vi "test_vlp16.vi"() -> ()   [LabVIEW 2019]
uses:
  <vilib>/Utility/miscctls.llb/LV3DPointTypeDef.ctl
  <vilib>/picture/3D Picture Control/Object/Create Object (drawable).vi
  <vilib>/picture/3D Picture Control/Object/Add Object (no reference).vi
  <vilib>/picture/3D Picture Control/Helpers/Set Light (no reference).vi
  <vilib>/picture/3D Picture Control/NI_3D Picture Control.lvlib
panel:
  in  "VLP16 cfg":T1={"h range"={82, -88}, "v range"={7, -9}} {"v range" scale=-15.0..15.0; "h range" scale=-180.0..180.0}
  in  "탭 컨트롤":enum32{"xy graph", "Data"}(tab)
  out "size_vlp-array":i32=12936
  out "3D Picture":refnum<vi>(3d-picture)
  in  "Draw Mode":T2(ring)
  in  "Size":dbl(slide)=1.3265306122448979 scale=0.0..10.0
  out "frame per s":dbl=9.75287984411405 format="%#_2g"
  out "For loop":i32=76
  in  "N of slice":u32=2048
  in  "dt":u32=10
  in  "Enable 3D":bool
  out "XY data":cluster{"x":dbl, "y":dbl}[](graph)
  in  "limit":dbl(slide) scale=0.0..10.0
  out "all_data":T3(array[cluster])
  out "xyz data":cluster{"x":dbl, "y":dbl, "z":dbl}[](array[cluster])
  in  "sel arrary":dbl[](array[numeric])=[-15.0, 1.0, -13.0, 3.0, -11.0, 5.0, -9.0, 7.0, -7.0, 9.0, -5.0, 11.0, -3.0, 13.0, -1.0, 15.0]
  in  "Enable deg":bool[](array[boolean])=[FALSE, TRUE, FALSE, TRUE, FALSE, TRUE, FALSE, FALSE, TRUE, FALSE, TRUE, FALSE, TRUE, FALSE, TRUE, FALSE]
  out "XY Graph":T4(graph)
  out "dt":u32=60
  out "Slide":i16(slide) scale=0.0..1000.0
  in  "stop":bool=TRUE
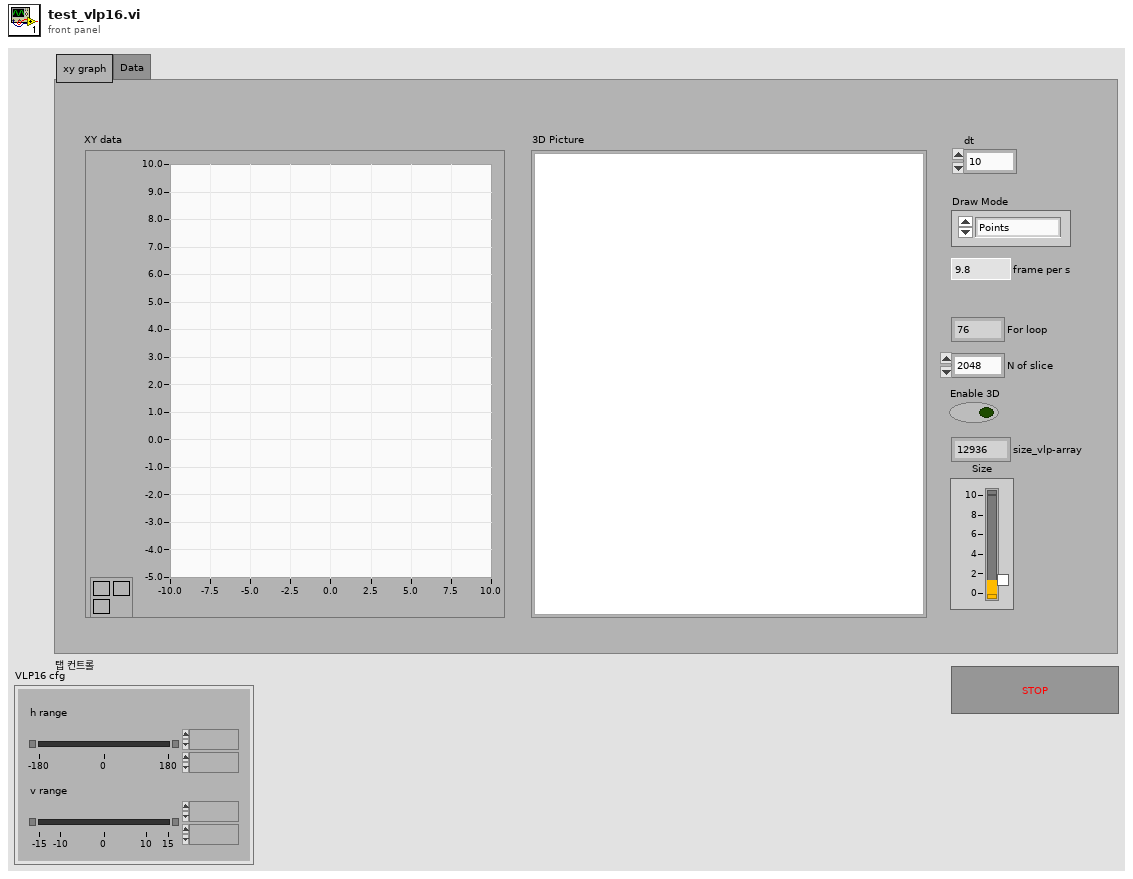
[diagram p1: front panel]
types:
  T1 = cluster{"h range":cluster{i16, i16}, "v range":cluster{i8, i8}}
  T2 = enum16{"Points", "Lines", "Line Strip", "Line Loop", "Triangles", "Triangle Strip", "Triangle Fan", "Quads", "Quad Strip", "Polygon"}
  T3 = cluster{"id":i32, "arimuth(degree)":dbl, "vertical(degree)":dbl, "distance(meter)":dbl, "reflectivity":u8, "times(s)":ext, "x":dbl, "y":dbl, "z":dbl}[]
  T4 = cluster{"Array out":cluster{"x":dbl, "y":dbl}[]}[]
  T5 = enum16{"Inherit Value", "Points", "Wireframe", "Polygons"}
  T6 = typedef "LV3DPointTypeDef.ctl" = cluster{"X":sgl, "Y":sgl, "Z":sgl}
  T7 = cluster{"id":i32, "azimuth(degree)":dbl, "vertical(degree)":dbl, "distance(meter)":dbl, "reflectivity":u8, "time(s)":ext, "x":dbl, "y":dbl, "z":dbl}
  T8 = cluster{"id":i32, "azimuth(degree)":dbl, "vertical(degree)":dbl, "distance(meter)":dbl, "reflectivity":u8, "time(s)":ext, "x":dbl, "y":dbl, "z":dbl}[]
  T9 = cluster{"limit inrange xydata":cluster{"x":dbl, "y":dbl}[]}
  T10 = cluster{"limit inrange xydata":cluster{"x":dbl, "y":dbl}[]}[]
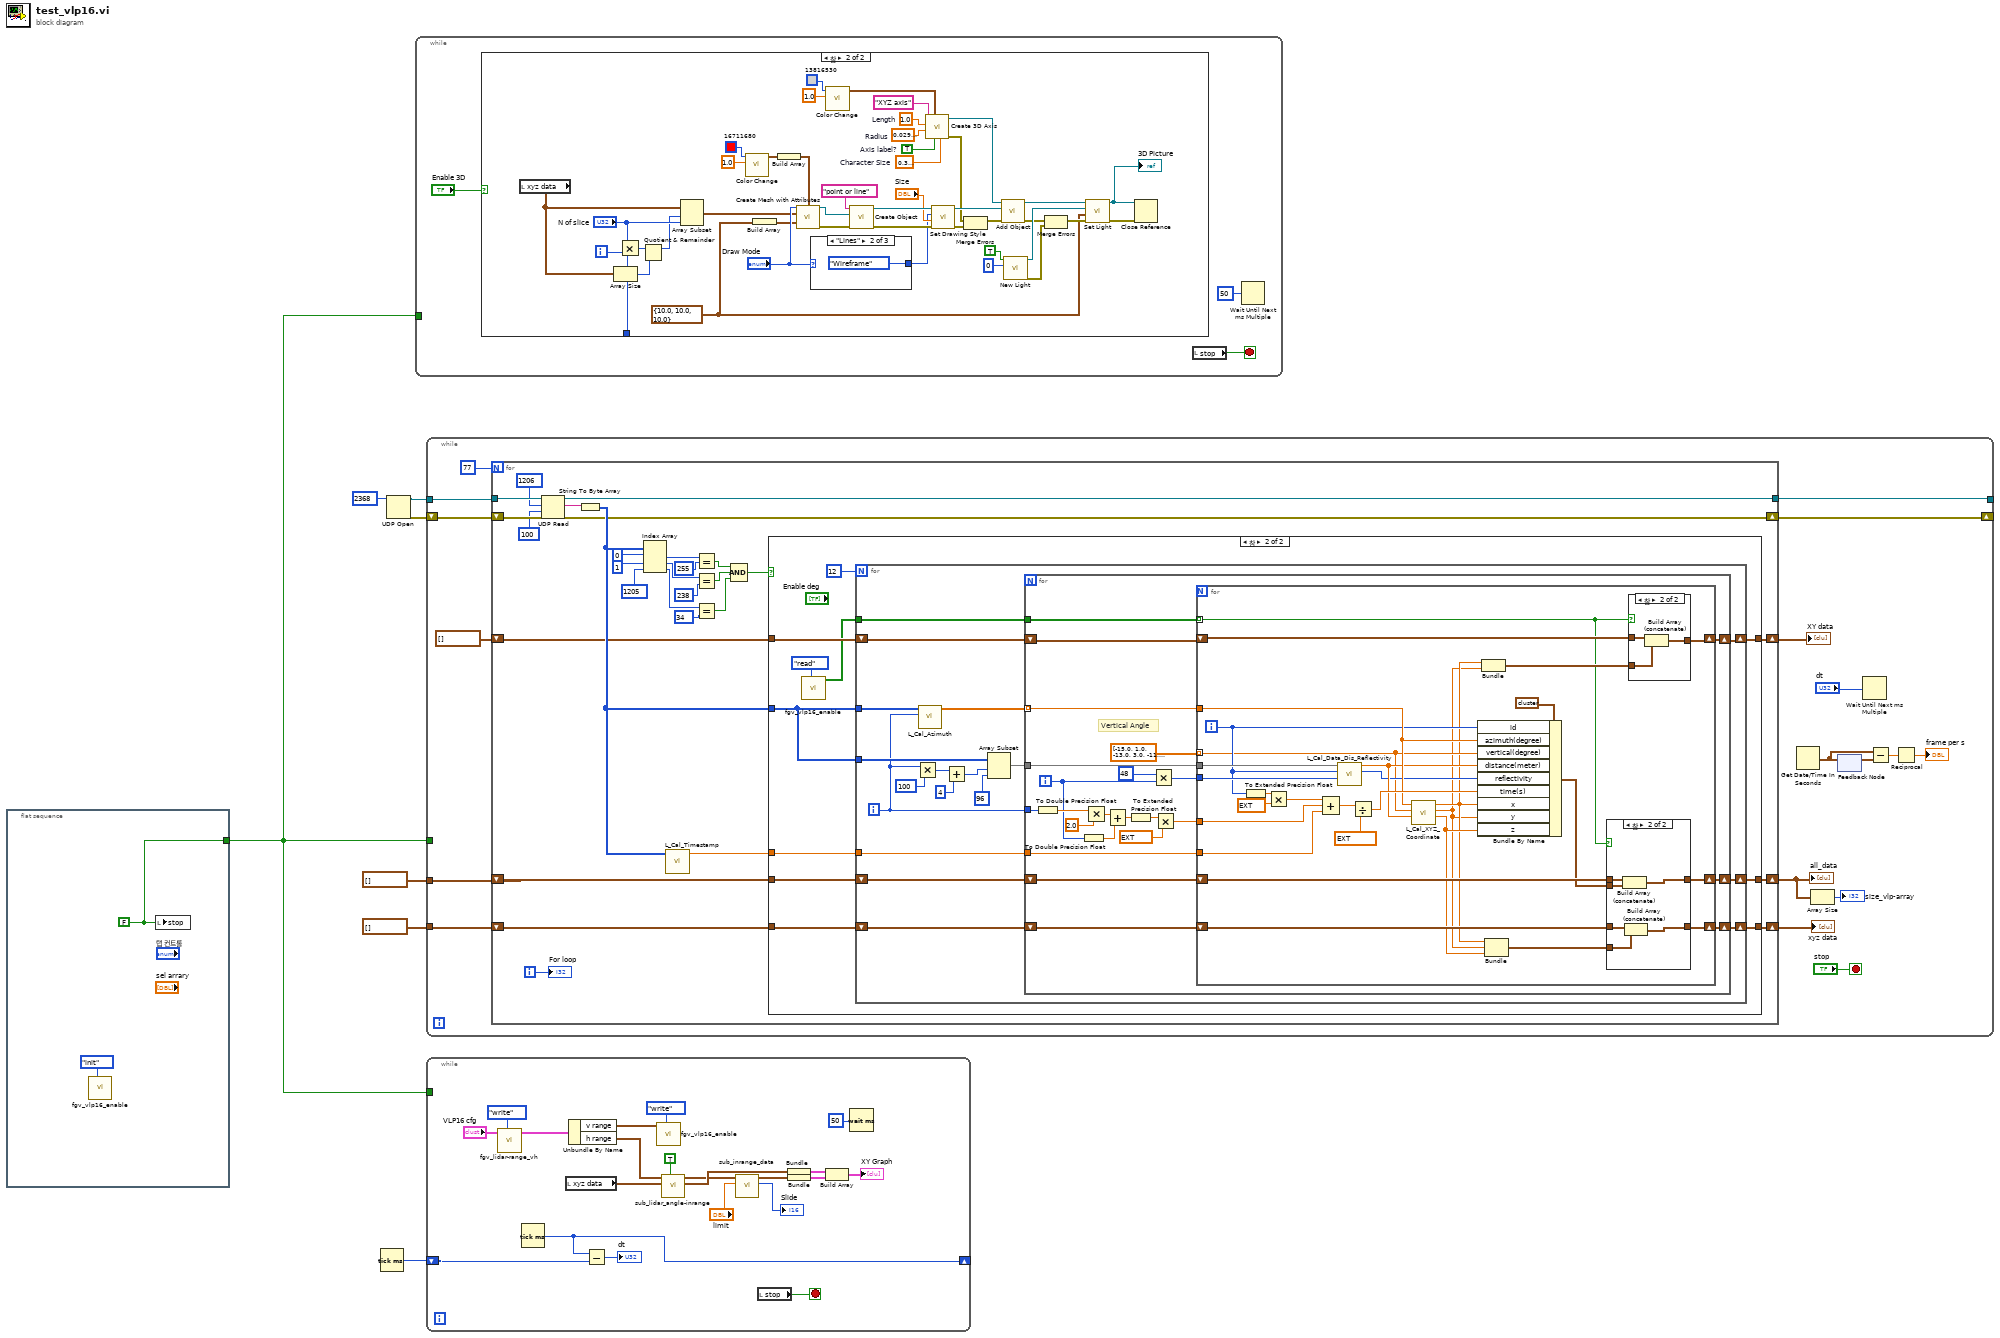
[diagram p0: block diagram]
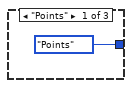
[diagram p3: hidden frame]
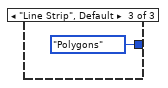
[diagram p4: hidden frame]
diagram:
  n1 = flat-sequence {
    tunnel: [w9] -> w1
    frame #0 {
      w9 = FALSE ("stop")
      n2 = call "fgv_vlp16_enable.vi"("cmd"=enum16{"init", "read", "write"}."init") -> ()  [unwired: 10 in, 1 out]
      n3 = local write "stop"(w9) -> ()
    }
  }
  n4 = Tick Count (ms)() -> (millisecond timer value=w2:u32)
  n5 = UDP Open(11:u16 2368 ("port")) -> (port=w5:refnum<k16>, 0:w4:errorcluster)  [unwired: 4 in, 1 out]
  n6 = while {
    tunnel: w1 -> [_]
    i -> [w12]
    stop <- w13 stop-if-true
    n7 = case shown="참" "Enable 3D" {
      tunnel: w12 -> [_ w14]
      frame False {
      }
      frame True {
        w25 = sgl 0.3  # Character Size
        w24 = T6 {"X"=10.0, "Y"=10.0, "Z"=10.0} ("Position")
        w44 = sgl 1.0  # Length
        w48 = sgl 0.03  # Radius
        w49 = TRUE  # Axis label?
        n8 = local read "xyz data"() -> (w16:cluster{"x":dbl, "y":dbl, "z":dbl}[])
        n9 = Array Size(array=w16) -> (size(s)=w18:i32)
        n10 = Multiply(x="N of slice", y=w14) -> (x*y=w19:u32)
        n11 = Quotient & Remainder(x=w19, y=w18) -> (x-y*floor(x/y)=w17:u32)  [unwired: 1 out]
        n12 = Array Subset(array=w16, index=w17, length="N of slice") -> (w15:cluster{"x":dbl, "y":dbl, "z":dbl}[])
        n13 = call <vilib>:"Color Change.vi"("Alpha"=1.0, "Color"=u32 16711680) -> ("RGBA"=w53:cluster{"R":sgl, "G":sgl, "B":sgl, "A":sgl})  [unwired: 9 in]
        n14 = Build Array(w24) -> (w23:T6[])
        n15 = Build Array(w53) -> (w52:cluster{"R":sgl, "G":sgl, "B":sgl, "A":sgl}[])
        n16 = call <vilib>:"Create Mesh with Attributes.vi"("Draw Mode"="Draw Mode", "Color Array"=w52, "Vertex Array"=w15, "Normal Array"=w23) -> ("New Mesh Refnum"=w56:refnum<vi>, "error out"=w55:errorcluster)  [unwired: 10 in]
        n17 = case shown="\"Lines\"" "Draw Mode" {
          tunnel: [T5."Points" ("Mode") T5."Wireframe" ("Mode") T5."Polygons" ("Mode")] -> w26
          frame "Points" {
          }
          frame "Lines" {
          }
          frame "Line Strip", Default {
          }
        }
        n18 = call <vilib>:"Color Change.vi"("Alpha"=1.0, "Color"=u32 13816530) -> ("RGBA"=w45:cluster{"R":sgl, "G":sgl, "B":sgl, "A":sgl})  [unwired: 9 in]
        n19 = call-poly <vilib>:"Create Object.vi"("error in (no error)"=w55, "Geometry"=w56, "Name"="point or line") -> ("error out"=w37:errorcluster, "Scene:New Object"=w39:refnum<vi>)  [unwired: 7 in]
        n20 = call <vilib>:"Create 3D Axis.vi"("Character Size"=w25, "Axis label?"=w49, "Color"=w45, "Radius"=w48, "Length"=w44, "Name"="XYZ axis") -> ("error out"=w31:errorcluster, "New Object Refnum"=w32:refnum<vi>)  [unwired: 4 in]
        n21 = call <vilib>:"Set Drawing Style.vi"("error in (no error)"=w37, "Size"="Size", "Mode"=w26, "Scene Object In"=w39) -> ("error out"=w36:errorcluster, "Scene Object Out"=w38:refnum<vi>)  [unwired: 6 in]
        n22 = Merge Errors(w31, w36) -> (w34:errorcluster)
        n23 = call-poly <vilib>:"Add Object.vi"("error in (no error)"=w34, "New Object In"=w38, "Scene Object In"=w32) -> ("error out"=w30:errorcluster, "Scene Object Out"=w43:refnum<vi>)  [unwired: 7 in]
        n24 = call <vilib>:"New Light.vi"("Light Number"=0, "At Infinity"=TRUE) -> ("error out"=w28:errorcluster, "New Light Refnum"=w42:refnum<vi>)  [unwired: 8 in]
        n25 = Merge Errors(w30, w28) -> (w29:errorcluster)
        n26 = call-poly <vilib>:"Set Light.vi"("error in (no error)"=w29, "Position"=w24, "Light Refnum In"=w42, "Scene Object In"=w43) -> ("error out"=w22:errorcluster, "Scene Object Out"=w21:refnum<vi>)  [unwired: 6 in]
        "3D Picture" <- w21
        n27 = Close Reference(reference=w21, error in (no error)=w22) -> ()  [unwired: 1 out]
      }
    }
    n28 = local read "stop"() -> (w13:bool)
    n29 = Wait Until Next ms Multiple(millisecond multiple=u32 50) -> ()  [unwired: 1 out]
  }
  n30 = while {
    shift-right: [w75] -> _
    shift-left: w4 -> [w76]
    tunnel: T3 [] -> [w74]
    tunnel: w5 -> [w77]
    tunnel: [w71] -> _
    tunnel: cluster{"x":dbl, "y":dbl, "z":dbl}[] [] -> [w65]
    tunnel: w1 -> [_]
    stop <- "stop" stop-if-true
    n31 = for {
      N: 77 -> [_]
      shift-right: [w86] -> w75
      shift-left: w76 -> [w89]
      shift-right: [w93] -> w62
      shift-left: w74 -> [w92]
      tunnel: w77 -> [w90]
      tunnel: [w85] -> w71
      shift-right: [w82] -> w63
      shift-left: w65 -> [w83]
      shift-right: [w78] -> w60
      shift-left: cluster{"x":dbl, "y":dbl}[] [] -> [w79]
      i -> [w81]
      n32 = UDP Read(connection ID=w90, max size (548)=1206, timeout ms (25000)=100, 8:w89) -> (data out=w88:string, error out=w86:errorcluster, 3:w85:refnum<k16>)  [unwired: 2 out]
      n33 = String To Byte Array(string=w88) -> (unsigned byte array=w87:u8[])
      n34 = Index Array(array=w87, index #1=0 ("index"), index #2=1 ("index"), index #3=1205 ("index")) -> (element #1=w103:u8, element #2=w100:u8, element #3=w98:u8)
      n35 = call "L_Cal_Timestamp.vi"("data"=w87) -> ("Timestamp"=w94:ext)  [unwired: 10 in]
      n36 = Equal?(x=w103, y=u8 255) -> (x = y?=w97:bool)
      n37 = Equal?(x=w100, y=u8 238) -> (x = y?=w96:bool)
      n38 = Equal?(x=w98, y=u8 34) -> (x = y?=w95:bool)
      n39 = Compound Arithmetic op=AND(w97, w96, w95) -> (w91:bool)
      n40 = case shown="참" w91 {
        tunnel: w94 -> [_ w120]
        tunnel: w87 -> [_ w119]
        tunnel: [w109 w118] -> w93
        tunnel: w92 -> [w109 w117]
        tunnel: w83 -> [w108 w115]
        tunnel: [w108 w114] -> w82
        tunnel: w79 -> [w107 w113]
        tunnel: [w107 w112] -> w78
        frame False {
        }
        frame True {
          n41 = call "fgv_vlp16_enable.vi"("cmd"=enum16{"init", "read", "write"}."read") -> ("Enable vlp ch out"=w110:bool[])  [unwired: 10 in]
          n42 = for {
            N: 12 -> [_]
            tunnel: w119 -> [w138]
            tunnel: w120 -> [w128]
            tunnel: w119 -> [w133]
            shift-right: [w126] -> w118
            shift-left: w117 -> [w127]
            shift-right: [w124] -> w114
            shift-left: w115 -> [w125]
            shift-right: [w122] -> w112
            shift-left: w113 -> [w123]
            tunnel: w110 -> [w121]
            i -> [w129]
            n43 = Multiply(x=w129, y=100) -> (x*y=w130:i32)
            n44 = call "L_Cal_Azimuth.vi"("DataBlock(-1)"=w129, "data"=w138) -> ("Azimuth(0,1)"=w137:dbl[])  [unwired: 9 in]
            n45 = Add(x=w130, y=4) -> (x+y=w135:i32)
            n46 = Array Subset(array=w133, index=w135, length=96 ("index")) -> (w132:u8[])
            n47 = for {
              tunnel: w137 -> [w151] mode=indexing
              tunnel: w132 -> [w161]
              tunnel: w129 -> [w148]
              tunnel: w128 -> [w152]
              shift-right: [w149] -> w126
              shift-left: w127 -> [w150]
              shift-right: [w143] -> w124
              shift-left: w125 -> [w144]
              shift-right: [w140] -> w122
              shift-left: w123 -> [w141]
              tunnel: w121 -> [w139]
              i -> [w145]
              # "Vertical Angle"
              n48 = To Double Precision Float(number=w148) -> (double precision float=w147:dbl)
              n49 = To Double Precision Float(number=w145) -> (double precision float=w146:dbl)
              n50 = Multiply(x=w147, y=2.0) -> (x*y=w156:dbl)
              n51 = Add(x=w156, y=w146) -> (x+y=w157:dbl)
              n52 = To Extended Precision Float(1:w157) -> (0:w158:ext)
              n53 = Multiply(x=48, y=w145) -> (x*y=w159:i32)
              n54 = Multiply(x=w158, y=ext 55.296) -> (x*y=w153:ext)
              n55 = for {
                tunnel: w161 -> [w190]
                tunnel: w159 -> [w189]
                tunnel: w153 -> [w185]
                tunnel: w152 -> [w184]
                tunnel: w151 -> [w179]
                shift-right: [w174] -> w149
                shift-left: w150 -> [w177]
                shift-right: [w171] -> w143
                shift-left: w144 -> [w172]
                tunnel: dbl[] [-15.0, 1.0, -13.0, 3.0, -11.0, 5.0, -9.0, 7.0, -7.0, 9.0, -5.0, 11.0, -3.0, 13.0, -1.0, 15.0] -> [w168] mode=indexing
                shift-right: [w163] -> w140
                shift-left: w141 -> [w164]
                tunnel: w139 -> [w162] mode=indexing
                i -> [w175]
                n56 = To Extended Precision Float(1:w175) -> (0:w188:ext)
                n57 = Multiply(x=w188, y=ext 2.304) -> (x*y=w186:ext)
                n58 = Compound Arithmetic op=ADD(w186, w185, w184) -> (w182:ext)
                n59 = call "L_Cal_Data_Dis_Reflectivity.vi"("Index(0 or 1)"=w189, "ID"=w175, "data"=w190) -> ("reflectivity"=w176:u8, "Distance"=w178:dbl)  [unwired: 7 in]
                n60 = Divide(x=w182, y=ext 1000000.0) -> (x/y=w180:ext)
                n61 = call "L_Cal_XYZ_Coordinate.vi"("distance"=w178, "vertical"=w168, "azimuth"=w179) -> ("z"=w170:dbl, "y"=w166:dbl, "x"=w167:dbl)  [unwired: 6 in]
                n62 = Bundle By Name(cluster=T7 {"id"=0, "azimuth(degree)"=0.0, "vertical(degree)"=0.0, "distance(meter)"=0.0, "reflectivity"=0, "time(s)"=0.0, "x"=0.0, "y"=0.0, "z"=0.0}, "id"=w175, "azimuth(degree)"=w179, "vertical(degree)"=w168, "distance(meter)"=w178, "reflectivity"=w176, "time(s)"=w180, "x"=w167, "y"=w166, "z"=w170) -> (w173:T7)
                n63 = Bundle("x"=w167, "y"=w166) -> (w165:cluster{"x":dbl, "y":dbl})  [unwired: 1 in]
                n64 = Bundle("x"=w167, "y"=w166, "z"=w170) -> (w169:cluster{"x":dbl, "y":dbl, "z":dbl})  [unwired: 1 in]
                n65 = case shown="참" w162 {
                  tunnel: w177 -> [w192 w198]
                  tunnel: [w192 w197] -> w174
                  tunnel: w173 -> [_ w196]
                  tunnel: w172 -> [w191 w195]
                  tunnel: [w191 w194] -> w171
                  tunnel: w169 -> [_ w193]
                  frame False {
                  }
                  frame True {
                    n66 = Build Array (concatenate)(w198, w196) -> (w197:T8)
                    n67 = Build Array (concatenate)(w195, w193) -> (w194:cluster{"x":dbl, "y":dbl, "z":dbl}[])
                  }
                }
                n68 = case shown="참" w162 {
                  tunnel: w165 -> [_ w202]
                  tunnel: w164 -> [w199 w201]
                  tunnel: [w199 w200] -> w163
                  frame False {
                  }
                  frame True {
                    n69 = Build Array (concatenate)(w201, w202) -> (w200:cluster{"x":dbl, "y":dbl}[])
                  }
                }
              }
            }
          }
        }
      }
      "For loop" <- w81
    }
    "all_data" <- w62
    "xyz data" <- w63
    "XY data" <- w60
    n70 = Get Date/Time In Seconds() -> (seconds since 1Jan1904=w69:timestamp)
    n71 = Array Size(array=w62) -> (size(s)=→"size_vlp-array":i32)
    n72 = feedback #1() -> (w68:timestamp)  [unwired: 1 in]
    n73 = feedback-in #1(w69) -> ()
    n74 = Wait Until Next ms Multiple(millisecond multiple="dt") -> ()  [unwired: 1 out]
    n75 = Subtract(x=w69, y=w68) -> (x-y=w67:dbl)
    n76 = Reciprocal(x=w67) -> (1/x=→"frame per s":dbl)
  }
  n77 = while {
    shift-right: [w220] -> _
    shift-left: w2 -> [w221]
    tunnel: w1 -> [_]
    stop <- w222 stop-if-true
    n78 = call "fgv_lidar-range_vh.vi"("cmd"=enum16{"read", "write"}."write", "VLP16 cfg"="VLP16 cfg") -> ("VLP16 cfg out"=w213:T1)  [unwired: 9 in]
    n79 = Tick Count (ms)() -> (millisecond timer value=w220:u32)
    n80 = local read "xyz data"() -> (w206:cluster{"x":dbl, "y":dbl, "z":dbl}[])
    n81 = Unbundle By Name(w213) -> ("v range"=w217:cluster{i8, i8}, "h range"=w205:cluster{i16, i16})
    n82 = Subtract(x=w220, y=w221) -> (x-y=→"dt":u32)
    n83 = call "fgv_vlp16_enable.vi"("cmd"=enum16{"init", "read", "write"}."write", "v range"=w217) -> ()  [unwired: 9 in, 1 out]
    n84 = call "sub_lidar_angle-inrange.vi"("3d"=TRUE, "3D data"=w206, "h range"=w205) -> ("xydata"=w204:cluster{"x":dbl, "y":dbl}[], "Array out"=w203:cluster{"x":dbl, "y":dbl}[])  [unwired: 6 in, 1 out]
    n85 = call "sub_inrange_data.vi"("limit"="limit", "xy_lidar data"=w203) -> ("limit point out"=→"Slide":u16, "limit inrange xydata"=w208:cluster{"x":dbl, "y":dbl}[])  [unwired: 7 in, 1 out]
    n86 = local read "stop"() -> (w222:bool)
    n87 = Bundle("xydata"=w204) -> (w215:cluster{"xydata":cluster{"x":dbl, "y":dbl}[]})  [unwired: 1 in]
    n88 = Bundle("limit inrange xydata"=w208) -> (w214:T9)  [unwired: 1 in]
    n89 = Build Array(w215, w214) -> (→"XY Graph":T10)
    n90 = Wait (ms)(milliseconds to wait=u32 50) -> ()  [unwired: 1 out]
  }
